vi "Alazar_conTrig.vi"(3 "Voltage Scale":dbl(ring)=2.0 items=["8 V"=8.0, "4 V"=4.0, "2 V"=2.0, "800 mV"=0.8, "400 mV"=0.4, "200 mV"=0.2, "80 mV"=0.08], 4 "Trigger":T1 {"Coupling" items=["DC 1 MOhm", "AC 1 MOhm", "DC 50 Ohm", "AC 50 Ohm"]; "Slope" items=["Positive", "Negative"]; "Level" format="%.2f"; "Source" items=["Chan 1", "External"]}, 5 "Device In":u32) -> (2 "InstrumentID Out":u32)   [LabVIEW 2022 SP3]
uses:
  C:/AlazarTech/ATS-VI/6.2.0/ATS_ctl/Device_Ctrl.ctl
  C:/AlazarTech/ATS-VI/6.2.0/ATS_ctl/TriggerOperation.ctl
  C:/AlazarTech/ATS-VI/6.2.0/ATS_ctl/ATS_TriggerSource_4Ch.ctl
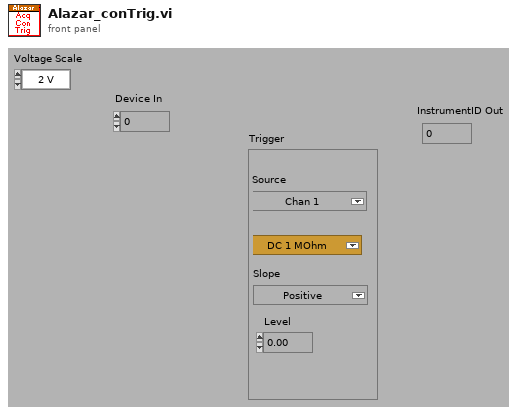
[diagram p1: front panel]
types:
  T1 = cluster{"Source":u16, "Coupling":u16, "Slope":u16, "Level":dbl}
  T2 = typedef "TriggerOperation.ctl" = enum16{"Only X", "Only Y", "X or Y", "X and Y", "X xor Y", "X and not Y", "not X and Y"}
  T3 = typedef "Device_Ctrl.ctl" = enum16{"Status", "About", "Arm", "ForceTrig", "Abort", "Initialize", "Init (NoPreset)", "Info", "Close", "Calibrate", "SetManually", "LED_ON", "LED_OFF"}
  T4 = typedef "ATS_TriggerSource_4Ch.ctl" = enum32{"Chan_A", "Chan_B", "External", "Disable", "Chan_C", "Chan_D"}
  T5 = typedef "Device_Info.ctl" = cluster{"Handle":u32, "Board":string, "CPLD":string, "MemorySize":u32, "SampleSize":u8, "ID":i32, "High_Memory":bool, "Chan/Board":u8}
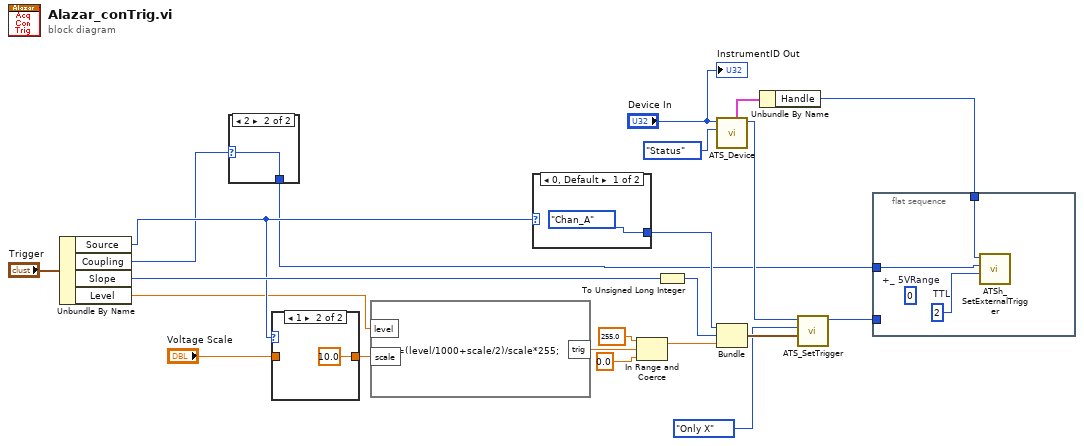
[diagram p0: block diagram]
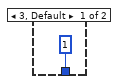
[diagram p2: hidden frame]
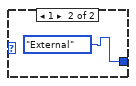
[diagram p4: hidden frame]
diagram:
  n1 = Unbundle By Name("Trigger") -> ("Source"=w11:u16, "Coupling"=w5:u16, "Slope"=w16:u16, "Level"=w10:dbl)
  n2 = case shown="2" w5 {
    selector: w5 -> [_ w24]
    tunnel: [u32 1 ("Coupling") w24] -> w4
    frame 3, Default {
    }
    frame 2 {
    }
  }
  n3 = case shown="1" w11 {
    tunnel: "Voltage Scale" -> [w25 _]
    tunnel: [w25 10.0 ("lower limit")] -> w9
    frame 0, Default {
    }
    frame 1 {
    }
  }
  n4 = formula code="trig=(level/1000+scale/2)/scale*255;"("level"=w10, "scale"=w9) -> ("trig"=w8:dbl)
  n5 = case shown="0, Default" w11 {
    tunnel: [ATS_TriggerSource_4Ch."Chan_A" ("Source") ATS_TriggerSource_4Ch."External" ("Source")] -> w15
    frame 0, Default {
    }
    frame 1 {
    }
  }
  n6 = In Range and Coerce(upper limit=255.0, x=w8, lower limit=0.0) -> (coerced(x)=w7:dbl)  [unwired: 1 out]
  n7 = To Unsigned Long Integer(number=w16) -> (unsigned 32bit integer=w14:u32)
  n8 = call "ATS_Device.vi"("DevCtrl"=Device_Ctrl."Status", "DeviceIn"="Device In") -> ("DeviceOut"=w17:i32, "DevInfo"=w19:T5)  [unwired: 3 in, 5 out]
  n9 = Bundle("Source"=w15, w14, "upper limit"=w7) -> (w3:cluster{"Source":T4, u32, "upper limit":dbl})  [unwired: 1 in]
  n10 = Unbundle By Name(w19) -> ("Handle"=w18:u32)
  n11 = call "ATS_SetTrigger.vi"("Engine X"=w3, "TrigOperation"=TriggerOperation."Only X", "DeviceIn"=w17) -> ("DeviceOut"=w1:i32)  [unwired: 7 in, 1 out]
  n12 = flat-sequence {
    tunnel: w18 -> [w31]
    tunnel: w4 -> [w30]
    tunnel: w1 -> [_]
    frame #0 {
      w29 = u32 2  # TTL
      (unwired) u32 0  # +_ 5VRange
      n13 = call "ATSh_SetExternalTrigger.vi"("Range"=w29, "Coupling"=w30, "Handle"=w31) -> ()  [unwired: 7 in, 2 out]
    }
  }
  "InstrumentID Out" <- "Device In"
